vi "TDMS chan to HDF5 (dbl).vi"(0 "tdms file":refnum<k34>, 1 "close dataset? (T)":bool=TRUE, 5 "group name in":string, 7 "channel name in":string, 11 "error in (no error)":errorcluster, 13 "HDF5 Ref":T1) -> (4 "tdms file out":refnum<k34>, 6 "group name out":string, 8 "channel name out":string, 10 "dataset out":T1, 15 "error out":errorcluster)   [LabVIEW 2012]
uses:
  <vilib>/addons/_hdf5/library.llb/HDF5 Ref.ctl
  <vilib>/addons/_hdf5/dataspace.llb/H5S_seloper_t.ctl
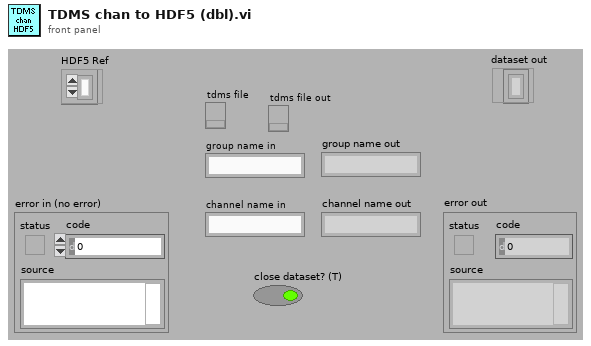
[diagram p1: front panel]
types:
  T1 = typedef "HDF5 Ref.ctl" = refnum<k1>
  T2 = typedef "H5S_seloper_t.ctl" = i32
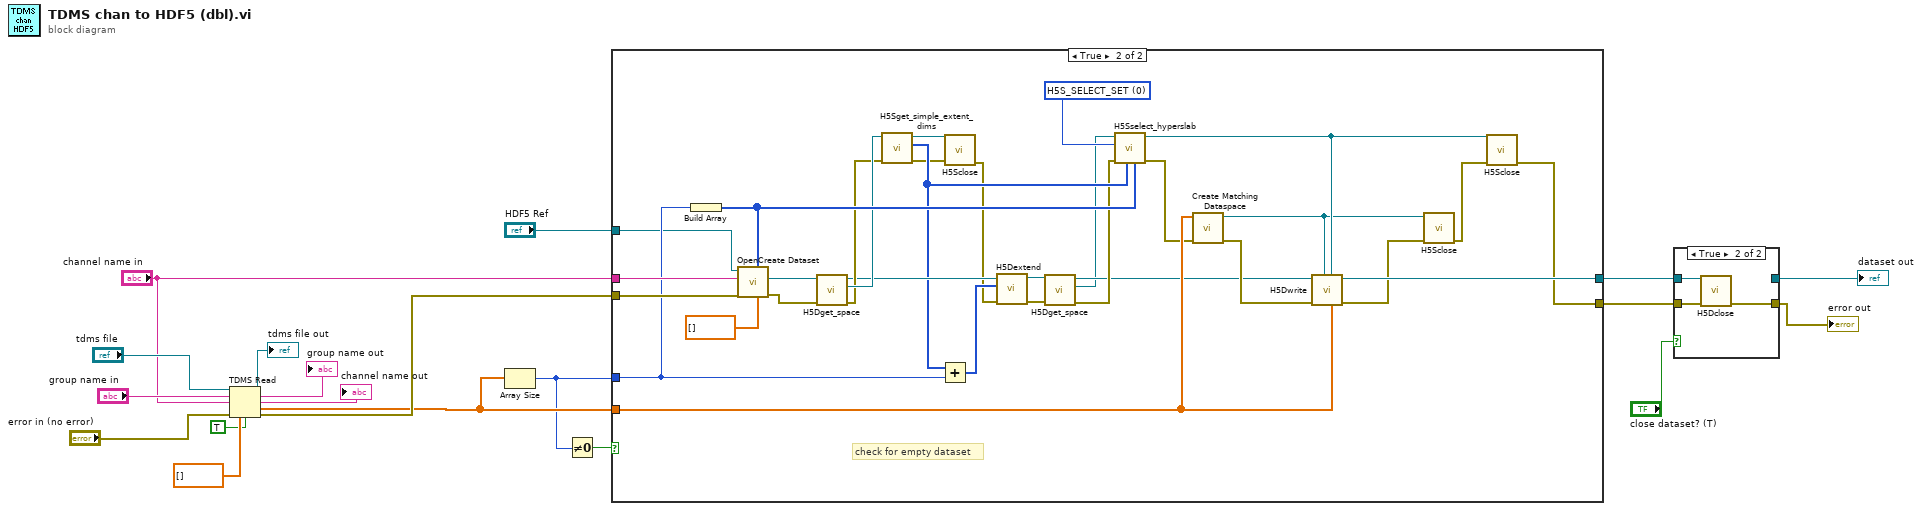
[diagram p0: block diagram]
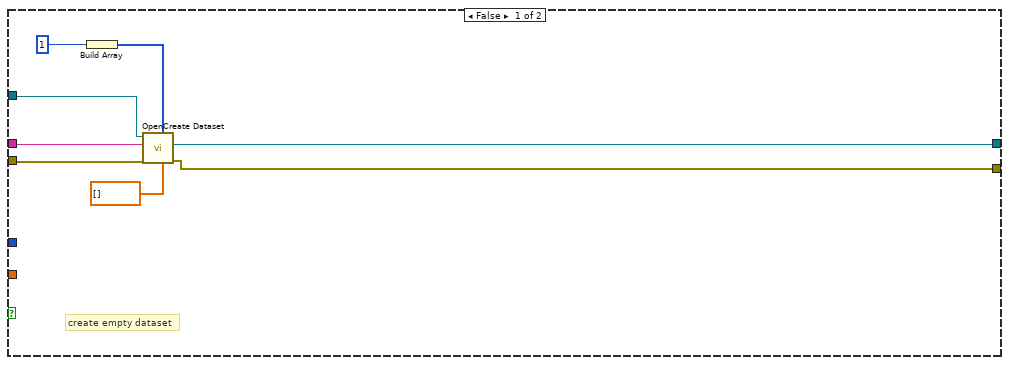
[diagram p2: hidden frame]
diagram:
  n1 = TDMS Read(0:"tdms file", 5:"group name in", 7:"channel name in", 11:"error in (no error)", 12:dbl[] [], 13:TRUE ("return channels in file order? (F)")) -> (4:→"tdms file out":refnum<k34>, 6:→"group name out":string, 8:→"channel name out":string, 10:w6:dbl[], 15:w15:errorcluster)  [unwired: 2 in, 1 out]
  n2 = Array Size(array=w6) -> (size(s)=w4:i32)
  n3 = Not Equal To 0?(x=w4) -> (x != 0?=w3:bool)
  n4 = case shown="True" w3 {
    tunnel: "channel name in" -> [w26 w58]
    tunnel: w15 -> [w25 w57]
    tunnel: [w22 w52] -> w10
    tunnel: [w23 w51] -> w9
    tunnel: w6 -> [_ w50]
    tunnel: w4 -> [_ w29]
    tunnel: "HDF5 Ref" -> [w24 w28]
    frame False {
      # "create empty dataset"
      n5 = Build Array(1) -> (w21:i32[])
      n6 = call "OpenCreate Dataset.vi"("Datatype"=dbl[] [], "Chunk size"=w21, "error in (no error)"=w25, "Dataset Path"=w26, "HDF5 Ref"=w24) -> ("error out"=w23:errorcluster, "HDF5 Dataset Ref out"=w22:T1)  [unwired: 4 in, 1 out]
    }
    frame True {
      w45 = T2 0 items=["H5S_SELECT_NOOP"=-1, "H5S_SELECT_SET"=0, "H5S_SELECT_OR"=1, "H5S_SELECT_AND"=2, "H5S_SELECT_XOR"=3, "H5S_SELECT_NOTB"=4, "H5S_SELECT_NOTA"=5, "H5S_SELECT_APPEND"=6, "H5S_SELECT_PREPEND"=7] ("Operator")
      # "check for empty dataset"
      n7 = Build Array(w29) -> (w53:i32[])
      n8 = call "OpenCreate Dataset.vi"("Datatype"=dbl[] [], "Chunk size"=w53, "error in (no error)"=w57, "Dataset Path"=w58, "HDF5 Ref"=w28) -> ("error out"=w56:errorcluster, "HDF5 Dataset Ref out"=w55:T1)  [unwired: 4 in, 1 out]
      n9 = call <vilib>:"H5Dget_space.vi"("error in (no error)"=w56, "HDF5 Dataset Ref"=w55) -> ("error out"=w48:errorcluster, "HDF5 Dataspace Ref"=w49:T1, "HDF5 Dataset Ref out"=w46:T1)  [unwired: 5 in]
      n10 = call <vilib>:"H5Sget_simple_extent_dims.vi"("error in (no error)"=w48, "HDF5 Space Ref"=w49) -> ("error out"=w41:errorcluster, "Dims"=w44:i32[], "HDF5 Ref out"=w40:T1)  [unwired: 4 in, 1 out]
      n11 = Add(x=w44, y=w29) -> (x+y=w47:i32[])
      n12 = call <vilib>:"H5Sclose.vi"("error in (no error)"=w41, "HDF5 Dataspace Ref"=w40) -> ("error out"=w37:errorcluster)  [unwired: 7 in]
      n13 = call <vilib>:"H5Dextend.vi"("error in (no error)"=w37, "Size"=w47, "HDF5 Dataset Ref"=w46) -> ("error out"=w38:errorcluster, "HDF5 Dataset Ref out"=w39:T1)  [unwired: 5 in]
      n14 = call <vilib>:"H5Dget_space.vi"("error in (no error)"=w38, "HDF5 Dataset Ref"=w39) -> ("error out"=w36:errorcluster, "HDF5 Dataspace Ref"=w34:T1, "HDF5 Dataset Ref out"=w35:T1)  [unwired: 5 in]
      n15 = call <vilib>:"H5Sselect_hyperslab.vi"("Count"=w53, "Start"=w44, "error in (no error)"=w36, "Operator"=w45, "HDF5 Space Ref"=w34) -> ("error out"=w43:errorcluster, "HDF5 Ref out"=w33:T1)  [unwired: 5 in]
      n16 = call <vilib>:"Create Matching Dataspace.vi"("error in (no error)"=w43, "Data"=w50) -> ("error out"=w42:errorcluster, "HDF5 Dataspace Ref"=w32:T1)  [unwired: 6 in]
      n17 = call <vilib>:"H5Dwrite.vi"("Variant"=w50, "HDF5 File Space Ref (H5S_ALL)"=w33, "HDF5 Memory Space Ref (H5S_ALL)"=w32, "error in (no error)"=w42, "HDF5 Dataset Ref"=w35) -> ("error out"=w31:errorcluster, "HDF5 Ref out"=w52:T1)  [unwired: 5 in]
      n18 = call <vilib>:"H5Sclose.vi"("error in (no error)"=w31, "HDF5 Dataspace Ref"=w32) -> ("error out"=w30:errorcluster)  [unwired: 7 in]
      n19 = call <vilib>:"H5Sclose.vi"("error in (no error)"=w30, "HDF5 Dataspace Ref"=w33) -> ("error out"=w51:errorcluster)  [unwired: 7 in]
    }
  }
  n20 = case shown="True" "close dataset? (T)" {
    tunnel: w10 -> [w60 w63]
    tunnel: w9 -> [w59 w62]
    tunnel: [w59 w61] -> w5
    tunnel: [w60 _] -> w7
    frame False {
    }
    frame True {
      n21 = call <vilib>:"H5Dclose.vi"("error in (no error)"=w62, "HDF5 Dataset Ref"=w63) -> ("error out"=w61:errorcluster)  [unwired: 7 in]
    }
  }
  "dataset out" <- w7
  "error out" <- w5
